vi "Read Msg Input.vi"(11 "Stop Msg in":refnum<class "Stop Msg.lvclass">) -> (2 "Msg Input":refnum<class "Msg Input.lvclass">)   [LabVIEW 2025, in "jettl.lvlib" / "Stop jettl Msg.lvlib" / "Stop Msg.lvclass"]
uses:
  Stop Msg.lvclass
  Msg Input/Msg Input.lvclass
  Stop Msg.lvclass/Stop Msg.ctl
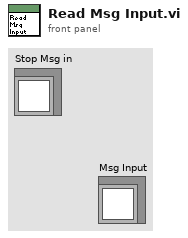
[diagram p1: front panel]
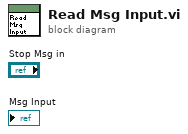
[diagram p0: block diagram]
diagram:
